vi "34461.vi"() -> ()   [LabVIEW 2014]
panel:
  out "波形图表":dbl[](graph)
  out "已采样数量":dbl
  in  "Range":dbl=-1.0 caption="Range (-1)" format="%.2p"
  in  "Absolute Resolution (1E-6)":dbl=1e-06 format="%.2p"
  in  "Measurement Function (DC Volts)":i32(ring)=1 items=["DC Volts"=1, "AC Volts"=2, "DC Current"=3, "AC Current"=4, "2 Wire Resistance"=5, "4 Wire Resistance"=101, "Frequency"=104, "Period"=105, "Temperature"=108, "Continuity"=1001, "Diode"=1002, "DC Volts Ratio"=1003, "Capacitance"=1004]
  in  "resource name":refnum<k15>
  in  "路径":path=path "test"
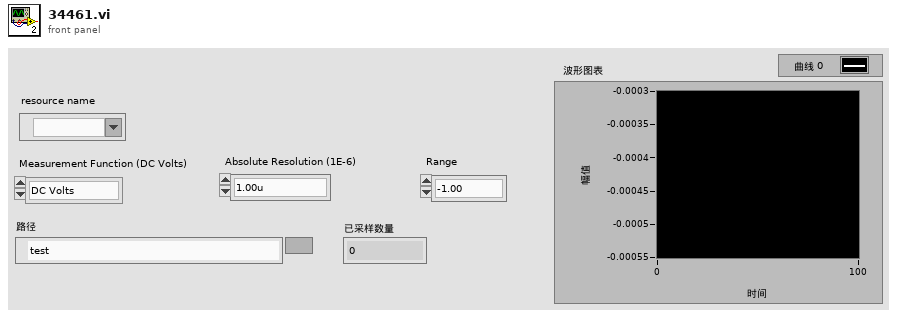
[diagram p1: front panel]
types:
  T1 = enum16{"open", "open or create", "create or replace", "create", "open (read-only)"}
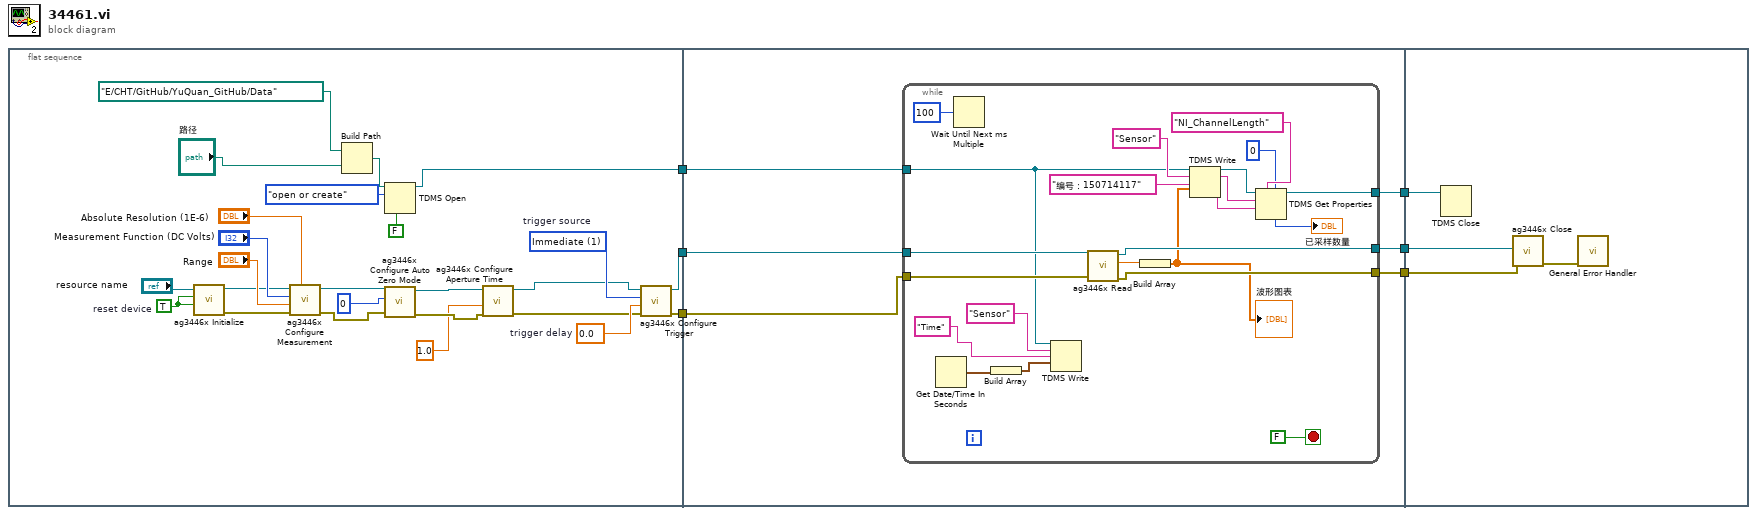
[diagram p0: block diagram]
diagram:
  n1 = flat-sequence {
    tunnel: [w13] -> w6
    tunnel: [w8] -> w5
    tunnel: [w7] -> w4
    tunnel: [w37] -> w3
    tunnel: [w36] -> w2
    tunnel: w6 -> [w35]
    tunnel: [w34] -> w1
    tunnel: w5 -> [w33]
    tunnel: w4 -> [w32]
    tunnel: w3 -> [w62]
    tunnel: w2 -> [w61]
    tunnel: w1 -> [w60]
    frame #0 {
      w11 = 0.0  # trigger delay
      w12 = 1 items=["Immediate"=1, "External"=2, "Software Trigger Function"=3, "GPIB Get"=101, "TTL0"=111, "TTL1"=112, "TTL2"=113, "TTL3"=114, "TTL4"=115, "TTL5"=116, "TTL6"=117, "TTL7"=118, "ECL0"=119, "ECL1"=120, "PXI Star"=131, "RTSI 0"=140, "RTSI 1"=141, "RTSI 2"=142, "RTSI 3"=143, "RTSI 4"=144, "RTSI 5"=145, "RTSI 6"=146]  # trigger source
      w20 = TRUE  # reset device
      n2 = call "ag3446x Initialize.vi"("Reset Device (Yes)"=w20, "ID Query (Yes)"=w20, "resource name"="resource name") -> ("error out"=w27:errorcluster, "instrument handle out"=w26:refnum<k15>)  [unwired: 7 in]
      n3 = call "ag3446x Configure Measurement.vi"("Absolute Resolution (1E-6)"="Absolute Resolution (1E-6)", "error in (no error)"=w27, "Range (-1)"="Range", "Measurement Function (DC Volts)"="Measurement Function (DC Volts)", "instrument handle"=w26) -> ("error out"=w23:errorcluster, "instrument handle out"=w25:refnum<k15>)  [unwired: 5 in]
      n4 = Build Path(base path=path "E:/CHT/GitHub/YuQuan_GitHub/Data", name or relative path="路径") -> (appended path=w17:path)
      n5 = TDMS Open(6:FALSE ("disable buffering (T)"), 10:T1."open or create" ("operation"), 11:w17) -> (3:w13:refnum<k34>)  [unwired: 4 in, 1 out]
      n6 = call <instrlib>:"ag3446x Configure Auto Zero Mode.vi"("error in (no error)"=w23, "Auto Zero Mode (On)"=0, "instrument handle"=w25) -> ("error out"=w21:errorcluster, "instrument handle out"=w22:refnum<k15>)  [unwired: 7 in]
      n7 = call <instrlib>:"ag3446x Configure Aperture Time.vi"("error in (no error)"=w21, "Aperture Time (10.0)"=1.0, "instrument handle"=w22) -> ("error out"=w9:errorcluster, "instrument handle out"=w10:refnum<k15>)  [unwired: 7 in]
      n8 = call "ag3446x Configure Trigger.vi"("error in (no error)"=w9, "Trigger Delay (0.0)"=w11, "Trigger Source (Immediate)"=w12, "instrument handle"=w10) -> ("error out"=w7:errorcluster, "instrument handle out"=w8:refnum<k15>)  [unwired: 6 in]
    }
    frame #1 {
      n9 = while {
        tunnel: w33 -> [w59]
        tunnel: w32 -> [w58]
        tunnel: [w57] -> w37
        tunnel: [w56] -> w36
        tunnel: w35 -> [w41]
        tunnel: [w46] -> w34
        stop <- FALSE stop-if-true
        n10 = Get Date/Time In Seconds() -> (seconds since 1Jan1904=w45:timestamp)
        n11 = Wait Until Next ms Multiple(millisecond multiple=100) -> ()  [unwired: 1 out]
        n12 = Build Array(w45) -> (w44:timestamp[])
        n13 = TDMS Write(0:w41, 5:"Sensor", 7:"Time", 9:w44) -> ()  [unwired: 2 in, 4 out]
        n14 = call "ag3446x Read.vi"("error in (no error)"=w58, "instrument handle"=w59) -> ("error out"=w57:errorcluster, "Reading"=w38:dbl, "instrument handle out"=w56:refnum<k15>)  [unwired: 7 in]
        n15 = Build Array(w38) -> (w39:dbl[])
        "波形图表" <- w39
        n16 = TDMS Write(0:w41, 5:"Sensor", 7:"编号：150714117", 9:w39) -> (4:w53:refnum<k34>, 6:w54:string, 8:w52:string)  [unwired: 2 in, 1 out]
        n17 = TDMS Get Properties(5:0, 7:"NI_ChannelLength", 9:w52, 10:w54, 11:w53) -> (3:w46:refnum<k34>, 4:→"已采样数量":i32)  [unwired: 1 in, 4 out]
      }
    }
    frame #2 {
      n18 = TDMS Close(11:w60) -> ()  [unwired: 1 in, 2 out]
      n19 = call "ag3446x Close.vi"("error in (no error)"=w62, "instrument handle"=w61) -> ("error out"=w63:errorcluster)  [unwired: 9 in]
      n20 = call <vilib>:"General Error Handler.vi"("error in (no error)"=w63) -> ()  [unwired: 2 in, 13 out]
    }
  }
